vi "Lab Panel V5.25.1.vi"() -> ()   [LabVIEW 2013] (continued)
                    n2215 = Unbundle By Name(w3901) -> ("1  (A) cal"=w3894:dbl, "1 (V) cal"=w3893:dbl, "1 (PF) cal"=w3892:dbl, "2 (A) cal"=w3891:dbl, "2 (V) cal"=w3890:dbl, "2 (PF) cal"=w3889:dbl)  [unwired: 4 out]
                    n2216 = Multiply(x=w3900, y=w3894) -> (x*y=w3887:dbl)
                    n2217 = Multiply(x=w3899, y=w3893) -> (x*y=w3881:dbl)
                    n2218 = Multiply(x=w3898, y=w3892) -> (x*y=w3886:dbl)
                    n2219 = Multiply(x=w3897, y=w3891) -> (x*y=w3884:dbl)
                    n2220 = Multiply(x=w3896, y=w3890) -> (x*y=w3883:dbl)
                    n2221 = Multiply(x=w3895, y=w3889) -> (x*y=w3882:dbl)
                    n2222 = local read "SIG LAB03-1"() -> (w3888:T2)
                    n2223 = local read "SIG LAB03-2"() -> (w3885:T2)
                    n2224 = Bundle By Name(cluster=w3888, "AMPS"=w3887, "VOLTS"=w3881, "PF"=w3886) -> (w3880:T2)
                    n2225 = Bundle By Name(cluster=w3885, "AMPS"=w3884, "VOLTS"=w3883, "PF"=w3882) -> (w3879:T2)
                    n2226 = global write "Global display 1.vi" "SIG LAB03-1"(w3880) -> ()
                    n2227 = global write "Global display 1.vi" "SIG LAB03-2"(w3879) -> ()
                    n2228 = local write "SIG LAB03-2"(w3879) -> ()
                    n2229 = local write "SIG LAB03-1"(w3880) -> ()
                  }
                  frame #5 {
                    n2230 = case shown="False" w3931 {
                      tunnel: [w3933 w3934] -> w3929
                      tunnel: w3930 -> [_ w3934]
                      frame False {
                        n2231 = local read "CAL LAB04"() -> (w3933:T14)
                      }
                      frame True {
                      }
                    }
                    n2232 = Unbundle By Name(w3932) -> ("OFF amps"=w3928:dbl, "VOLTS"=w3927:dbl, "PF"=w3926:dbl, "OFF amps"=w3925:dbl, "VOLTS"=w3924:dbl, "PF"=w3923:dbl)
                    n2233 = Unbundle By Name(w3929) -> ("1  (A) cal"=w3922:dbl, "1 (V) cal"=w3921:dbl, "1 (PF) cal"=w3920:dbl, "2 (A) cal"=w3919:dbl, "2 (V) cal"=w3918:dbl, "2 (PF) cal"=w3917:dbl)  [unwired: 4 out]
                    n2234 = Multiply(x=w3928, y=w3922) -> (x*y=w3915:dbl)
                    n2235 = Multiply(x=w3927, y=w3921) -> (x*y=w3914:dbl)
                    n2236 = Multiply(x=w3926, y=w3920) -> (x*y=w3913:dbl)
                    n2237 = Multiply(x=w3925, y=w3919) -> (x*y=w3911:dbl)
                    n2238 = Multiply(x=w3924, y=w3918) -> (x*y=w3910:dbl)
                    n2239 = Multiply(x=w3923, y=w3917) -> (x*y=w3909:dbl)
                    n2240 = local read "SIG LAB04-1"() -> (w3916:T2)
                    n2241 = local read "SIG LAB04-2"() -> (w3912:T2)
                    n2242 = Bundle By Name(cluster=w3916, "AMPS"=w3915, "VOLTS"=w3914, "PF"=w3913) -> (w3908:T2)
                    n2243 = Bundle By Name(cluster=w3912, "AMPS"=w3911, "VOLTS"=w3910, "PF"=w3909) -> (w3907:T2)
                    n2244 = global write "Global display 1.vi" "SIG LAB04-2"(w3907) -> ()
                    n2245 = global write "Global display 1.vi" "SIG LAB04-1"(w3908) -> ()
                    n2246 = local write "SIG LAB04-2"(w3907) -> ()
                    n2247 = local write "SIG LAB04-1"(w3908) -> ()
                  }
                  frame #6 {
                    n2248 = Unbundle By Name(w3960) -> ("OFF amps"=w3956:dbl, "VOLTS"=w3937:dbl, "PF"=w3955:dbl, "OFF amps"=w3954:dbl, "VOLTS"=w3953:dbl, "PF"=w3952:dbl)
                    n2249 = case shown="False" w3959 {
                      tunnel: [w3961 w3962] -> w3957
                      tunnel: w3958 -> [_ w3962]
                      frame False {
                        n2250 = local read "CAL LAB05"() -> (w3961:T14)
                      }
                      frame True {
                      }
                    }
                    n2251 = Unbundle By Name(w3957) -> ("1  (A) cal"=w3951:dbl, "1 (V) cal"=w3950:dbl, "1 (PF) cal"=w3949:dbl, "2 (A) cal"=w3948:dbl, "2 (V) cal"=w3947:dbl, "2 (PF) cal"=w3946:dbl)  [unwired: 4 out]
                    n2252 = Multiply(x=w3956, y=w3951) -> (x*y=w3944:dbl)
                    n2253 = Multiply(x=w3937, y=w3950) -> (x*y=w3943:dbl)
                    n2254 = Multiply(x=w3955, y=w3949) -> (x*y=w3942:dbl)
                    n2255 = Multiply(x=w3954, y=w3948) -> (x*y=w3940:dbl)
                    n2256 = Multiply(x=w3953, y=w3947) -> (x*y=w3939:dbl)
                    n2257 = Multiply(x=w3952, y=w3946) -> (x*y=w3938:dbl)
                    n2258 = local read "SIG LAB05-1"() -> (w3945:T2)
                    n2259 = local read "SIG LAB05-2"() -> (w3941:T2)
                    n2260 = Bundle By Name(cluster=w3945, "AMPS"=w3944, "VOLTS"=w3943, "PF"=w3942) -> (w3936:T2)
                    n2261 = Bundle By Name(cluster=w3941, "AMPS"=w3940, "VOLTS"=w3939, "PF"=w3938) -> (w3935:T2)
                    n2262 = global write "Global display 1.vi" "SIG LAB05-1"(w3936) -> ()
                    n2263 = global write "Global display 1.vi" "SIG LAB05-2"(w3935) -> ()
                    n2264 = local write "SIG LAB05-2"(w3935) -> ()
                    n2265 = local write "SIG LAB05-1"(w3936) -> ()
                  }
                  frame #7 {
                    n2266 = case shown="False" w3963 {
                      tunnel: w3965 -> [w3970 _]
                      tunnel: w3964 -> [w3969 _]
                      frame False {
                        # "update ambient referance temperature"
                        n2267 = case shown="True" w3970 {
                          tunnel: [w3972 100.0] -> w3971
                          frame False {
                            n2268 = local read "TEMP REF cal"() -> (w3972:dbl)
                          }
                          frame True {
                          }
                        }
                        n2269 = disable-structure shown="Disabled" {
                          frame Disabled {
                            n2270 = local read "Temp read loop"() -> ()  [unwired: 1 out]
                          }
                          frame Enabled {
                          }
                        }
                        n2271 = Multiply(x=w3971, y=w3969) -> (x*y=w3968:dbl)
                        n2272 = Subtract(x=w3968, y=272) -> (x-y=w3966:dbl)
                        "Amb Tp" <- w3966
                        n2273 = local write "Ref deg C"(w3966) -> ()
                        "deg C (volts)" <- w3969
                      }
                      frame True {
                      }
                    }
                  }
                }
              }
            }
          }
          frame #14 {
            # "save test data to file"
            n2274 = local read "on loops"() -> (w3993:dbl)
            n2275 = Get Date/Time In Seconds() -> (seconds since 1Jan1904=w3974:timestamp)
            "File Time Stamp" <- w3974
            n2276 = local read "jig cycle"() -> (w3990:dbl)
            n2277 = Format Date/Time String(time format string (%c)="%H:%M%:%S", seconds (now)=w3974) -> (date/time string=w3978:string)  [unwired: 1 in]
            n2278 = Add(x=w3993, y=4) -> (x+y=w3991:dbl)
            n2279 = Build Array(w3978) -> (w3977:string[])
            n2280 = Equal?(x=w3990, y=3) -> (x = y?=w3976:bool)
            n2281 = Equal?(x=w3990, y=w3991) -> (x = y?=w3975:bool)
            n2282 = stacked-sequence {
              tunnel: w3989 -> [w3999 _ _ _ _ _ _ _ _ _]
              tunnel: w3988 -> [_ w4075 _ _ _ _ _ _ _ _]
              tunnel: w3987 -> [_ _ w4155 _ _ _ _ _ _ _]
              tunnel: w3986 -> [_ _ _ w4235 _ _ _ _ _ _]
              tunnel: w3985 -> [_ _ _ _ w4315 _ _ _ _ _]
              tunnel: w3984 -> [_ _ _ _ _ w4395 _ _ _ _]
              tunnel: w3983 -> [_ _ _ _ _ _ w4475 _ _ _]
              tunnel: w3982 -> [_ _ _ _ _ _ _ w4555 _ _]
              tunnel: w3981 -> [_ _ _ _ _ _ _ _ w4635 _]
              tunnel: w3980 -> [_ _ _ _ _ _ _ _ _ w4715]
              tunnel: w3977 -> [w3998 w4079 w4159 w4239 w4319 w4399 w4479 w4559 w4639 w4719]
              tunnel: w3976 -> [w3997 w4078 w4158 w4238 w4318 w4398 w4478 w4558 w4638 w4718]
              tunnel: w3975 -> [w3996 w4077 w4157 w4237 w4317 w4397 w4477 w4557 w4637 w4717]
              tunnel: w3974 -> [w3995 w4076 w4156 w4236 w4316 w4396 w4476 w4556 w4636 w4716]
              frame #0 {
                n2283 = case shown="True" w3999 {
                  tunnel: w3998 -> [_ w4004]
                  tunnel: w3997 -> [_ w4003]
                  tunnel: w3996 -> [_ w4001]
                  tunnel: w3995 -> [_ w4000]
                  frame False {
                  }
                  frame True {
                    n2284 = local read "DISP LAB01-1"() -> (w4005:T4)
                    n2285 = local read "SIG LAB01-1"() -> (w4006:T2)
                    n2286 = local read "ON L01-1"() -> (w4002:cluster{"amps":dbl, "volts":dbl, "pf":dbl})
                    n2287 = Unbundle(w4006) -> ("AMPS"=w4012:dbl, "VOLTS"=w4010:dbl, "PF"=w4009:dbl, "Tmp Live"=w4008:dbl, "Tmp Neut"=w4011:dbl)
                    n2288 = Unbundle(w4005) -> ("CYCLE"=w4007:dbl)  [unwired: 2 out]
                    n2289 = stacked-sequence {
                      tunnel: w4012 -> [w4016 w4035]
                      tunnel: w4011 -> [_ w4034]
                      tunnel: w4010 -> [w4015 w4033]
                      tunnel: w4009 -> [w4014 w4032]
                      tunnel: w4008 -> [_ w4031]
                      tunnel: w4007 -> [_ w4030]
                      tunnel: w4004 -> [_ w4029]
                      tunnel: w4003 -> [w4017 _]
                      tunnel: w4002 -> [w4013 w4027]
                      tunnel: w4001 -> [_ w4028]
                      tunnel: w4000 -> [_ w4023]
                      frame #0 {
                        n2290 = case shown="True" w4017 {
                          tunnel: w4016 -> [_ w4022]
                          tunnel: w4015 -> [_ w4021]
                          tunnel: w4014 -> [_ w4020]
                          tunnel: w4013 -> [_ w4018]
                          frame False {
                          }
                          frame True {
                            n2291 = Bundle(cluster=w4018, "amps"=w4022, "volts"=w4021, "pf"=w4020) -> (w4019:cluster{"amps":dbl, "volts":dbl, "pf":dbl})
                            n2292 = local write "ON L01-1"(w4019) -> ()
                          }
                        }
                      }
                      frame #1 {
                        n2293 = Unbundle(w4027) -> ("amps"=w4026:dbl, "volts"=w4025:dbl, "pf"=w4024:dbl)
                        n2294 = case shown="True" w4028 {
                          tunnel: w4035 -> [_ w4036]
                          tunnel: w4034 -> [_ w4074]
                          tunnel: w4033 -> [_ _]
                          tunnel: w4032 -> [_ _]
                          tunnel: w4031 -> [_ w4073]
                          tunnel: w4030 -> [_ w4072]
                          tunnel: w4029 -> [_ w4040]
                          tunnel: w4026 -> [_ w4037]
                          tunnel: w4025 -> [_ w4069]
                          tunnel: w4024 -> [_ w4068]
                          tunnel: w4023 -> [_ w4038]
                          frame False {
                          }
                          frame True {
                            n2295 = local read "TDMS LAB01-1"() -> (w4071:refnum<k34>)
                            n2296 = Build Array(w4069) -> (w4065:dbl[])
                            n2297 = Build Array(w4068) -> (w4064:dbl[])
                            n2298 = Build Array(w4073) -> (w4063:dbl[])
                            n2299 = Build Array(w4074) -> (w4062:dbl[])
                            n2300 = Build Array(w4037) -> (w4067:dbl[])
                            n2301 = Build Array(w4036) -> (w4066:dbl[])
                            n2302 = Build Array(w4072) -> (w4061:dbl[])
                            n2303 = Build Array("AMPS ON", "AMPS OFF", "VOLTS", "PF", "TEMP Live", "TEMP Neut", "CYCLE") -> (w4045:string[])
                            n2304 = Bundle By Name("Y"=w4067, "t0"=w4038) -> (w4060:waveform(dbl))  [unwired: 1 in]
                            n2305 = Bundle By Name("Y"=w4066, "t0"=w4038) -> (w4059:waveform(dbl))  [unwired: 1 in]
                            n2306 = Bundle By Name("Y"=w4065, "t0"=w4038) -> (w4058:waveform(dbl))  [unwired: 1 in]
                            n2307 = Bundle By Name("Y"=w4064, "t0"=w4038) -> (w4057:waveform(dbl))  [unwired: 1 in]
                            n2308 = Bundle By Name("Y"=w4063, "t0"=w4038) -> (w4056:waveform(dbl))  [unwired: 1 in]
                            n2309 = Bundle By Name("Y"=w4062, "t0"=w4038) -> (w4055:waveform(dbl))  [unwired: 1 in]
                            n2310 = Bundle By Name("Y"=w4061, "t0"=w4038) -> (w4054:waveform(dbl))  [unwired: 1 in]
                            n2311 = Build Array(w4060, w4059, w4058, w4057, w4056, w4055, w4054) -> (w4053:waveform(dbl)[])
                            n2312 = TDMS Write(0:w4071, 5:"TEST VALUES", 7:w4045, 9:w4053) -> (4:w4044:refnum<k34>, 6:w4043:string, 15:w4042:errorcluster)  [unwired: 2 in, 1 out]
                            n2313 = TDMS Write(0:w4044, 5:w4043, 7:"TIME", 9:w4040, 11:w4042) -> (15:w4039:errorcluster)  [unwired: 1 in, 3 out]
                            n2314 = local write "data file error"(w4039) -> ()
                          }
                        }
                      }
                    }
                  }
                }
              }
              frame #1 {
                n2315 = case shown="True" w4075 {
                  tunnel: w4079 -> [_ w4084]
                  tunnel: w4078 -> [_ w4083]
                  tunnel: w4077 -> [_ w4081]
                  tunnel: w4076 -> [_ w4080]
                  frame False {
                  }
                  frame True {
                    n2316 = local read "DISP LAB01-2"() -> (w4085:T4)
                    n2317 = local read "SIG LAB01-2"() -> (w4086:T2)
                    n2318 = local read "ON L01-2"() -> (w4082:cluster{"amps":dbl, "volts":dbl, "pf":dbl})
                    n2319 = Unbundle(w4086) -> ("AMPS"=w4092:dbl, "VOLTS"=w4090:dbl, "PF"=w4089:dbl, "Tmp Live"=w4088:dbl, "Tmp Neut"=w4091:dbl)
                    n2320 = Unbundle(w4085) -> ("CYCLE"=w4087:dbl)  [unwired: 2 out]
                    n2321 = stacked-sequence {
                      tunnel: w4092 -> [w4096 w4115]
                      tunnel: w4091 -> [_ w4114]
                      tunnel: w4090 -> [w4095 w4113]
                      tunnel: w4089 -> [w4094 w4112]
                      tunnel: w4088 -> [_ w4111]
                      tunnel: w4087 -> [_ w4110]
                      tunnel: w4084 -> [_ w4109]
                      tunnel: w4083 -> [w4097 _]
                      tunnel: w4082 -> [w4093 w4107]
                      tunnel: w4081 -> [_ w4108]
                      tunnel: w4080 -> [_ w4103]
                      frame #0 {
                        n2322 = case shown="True" w4097 {
                          tunnel: w4096 -> [_ w4102]
                          tunnel: w4095 -> [_ w4101]
                          tunnel: w4094 -> [_ w4100]
                          tunnel: w4093 -> [_ w4098]
                          frame False {
                          }
                          frame True {
                            n2323 = Bundle(cluster=w4098, "amps"=w4102, "volts"=w4101, "pf"=w4100) -> (w4099:cluster{"amps":dbl, "volts":dbl, "pf":dbl})
                            n2324 = local write "ON L01-2"(w4099) -> ()
                          }
                        }
                      }
                      frame #1 {
                        n2325 = Unbundle(w4107) -> ("amps"=w4106:dbl, "volts"=w4105:dbl, "pf"=w4104:dbl)
                        n2326 = case shown="True" w4108 {
                          tunnel: w4115 -> [_ w4147]
                          tunnel: w4114 -> [_ w4154]
                          tunnel: w4113 -> [_ _]
                          tunnel: w4112 -> [_ _]
                          tunnel: w4111 -> [_ w4153]
                          tunnel: w4110 -> [_ w4152]
                          tunnel: w4109 -> [_ w4117]
                          tunnel: w4106 -> [_ w4149]
                          tunnel: w4105 -> [_ w4148]
                          tunnel: w4104 -> [_ w4146]
                          tunnel: w4103 -> [_ w4138]
                          frame False {
                          }
                          frame True {
                            n2327 = local read "TDMS LAB01-2"() -> (w4151:refnum<k34>)
                            n2328 = Build Array(w4148) -> (w4143:dbl[])
                            n2329 = Build Array(w4146) -> (w4142:dbl[])
                            n2330 = Build Array(w4153) -> (w4141:dbl[])
                            n2331 = Build Array(w4154) -> (w4140:dbl[])
                            n2332 = Build Array(w4149) -> (w4145:dbl[])
                            n2333 = Build Array(w4147) -> (w4144:dbl[])
                            n2334 = Build Array(w4152) -> (w4139:dbl[])
                            n2335 = Build Array("AMPS ON", "AMPS OFF", "VOLTS", "PF", "TEMP Live", "TEMP Neut", "CYCLE") -> (w4122:string[])
                            n2336 = Bundle By Name("Y"=w4145, "t0"=w4138) -> (w4137:waveform(dbl))  [unwired: 1 in]
                            n2337 = Bundle By Name("Y"=w4144, "t0"=w4138) -> (w4136:waveform(dbl))  [unwired: 1 in]
                            n2338 = Bundle By Name("Y"=w4143, "t0"=w4138) -> (w4135:waveform(dbl))  [unwired: 1 in]
                            n2339 = Bundle By Name("Y"=w4142, "t0"=w4138) -> (w4134:waveform(dbl))  [unwired: 1 in]
                            n2340 = Bundle By Name("Y"=w4141, "t0"=w4138) -> (w4133:waveform(dbl))  [unwired: 1 in]
                            n2341 = Bundle By Name("Y"=w4140, "t0"=w4138) -> (w4132:waveform(dbl))  [unwired: 1 in]
                            n2342 = Bundle By Name("Y"=w4139, "t0"=w4138) -> (w4131:waveform(dbl))  [unwired: 1 in]
                            n2343 = Build Array(w4137, w4136, w4135, w4134, w4133, w4132, w4131) -> (w4130:waveform(dbl)[])
                            n2344 = TDMS Write(0:w4151, 5:"TEST VALUES", 7:w4122, 9:w4130) -> (4:w4121:refnum<k34>, 6:w4120:string, 15:w4119:errorcluster)  [unwired: 2 in, 1 out]
                            n2345 = TDMS Write(0:w4121, 5:w4120, 7:"TIME", 9:w4117, 11:w4119) -> (15:w4116:errorcluster)  [unwired: 1 in, 3 out]
                            n2346 = local write "data file error"(w4116) -> ()
                          }
                        }
                      }
                    }
                  }
                }
              }
              frame #2 {
                n2347 = case shown="True" w4155 {
                  tunnel: w4159 -> [_ w4164]
                  tunnel: w4158 -> [_ w4163]
                  tunnel: w4157 -> [_ w4161]
                  tunnel: w4156 -> [_ w4160]
                  frame False {
                  }
                  frame True {
                    n2348 = local read "DISP LAB02-1"() -> (w4165:T4)
                    n2349 = local read "SIG LAB02-1"() -> (w4166:T2)
                    n2350 = local read "ON L02-1"() -> (w4162:cluster{"amps":dbl, "volts":dbl, "pf":dbl})
                    n2351 = Unbundle(w4166) -> ("AMPS"=w4172:dbl, "VOLTS"=w4170:dbl, "PF"=w4169:dbl, "Tmp Live"=w4168:dbl, "Tmp Neut"=w4171:dbl)
                    n2352 = Unbundle(w4165) -> ("CYCLE"=w4167:dbl)  [unwired: 2 out]
                    n2353 = stacked-sequence {
                      tunnel: w4172 -> [w4176 w4195]
                      tunnel: w4171 -> [_ w4194]
                      tunnel: w4170 -> [w4175 w4193]
                      tunnel: w4169 -> [w4174 w4192]
                      tunnel: w4168 -> [_ w4191]
                      tunnel: w4167 -> [_ w4190]
                      tunnel: w4164 -> [_ w4189]
                      tunnel: w4163 -> [w4177 _]
                      tunnel: w4162 -> [w4173 w4187]
                      tunnel: w4161 -> [_ w4188]
                      tunnel: w4160 -> [_ w4183]
                      frame #0 {
                        n2354 = case shown="True" w4177 {
                          tunnel: w4176 -> [_ w4182]
                          tunnel: w4175 -> [_ w4181]
                          tunnel: w4174 -> [_ w4180]
                          tunnel: w4173 -> [_ w4178]
                          frame False {
                          }
                          frame True {
                            n2355 = Bundle(cluster=w4178, "amps"=w4182, "volts"=w4181, "pf"=w4180) -> (w4179:cluster{"amps":dbl, "volts":dbl, "pf":dbl})
                            n2356 = local write "ON L02-1"(w4179) -> ()
                          }
                        }
                      }
                      frame #1 {
                        n2357 = Unbundle(w4187) -> ("amps"=w4186:dbl, "volts"=w4185:dbl, "pf"=w4184:dbl)
                        n2358 = case shown="True" w4188 {
                          tunnel: w4195 -> [_ w4227]
                          tunnel: w4194 -> [_ w4234]
                          tunnel: w4193 -> [_ _]
                          tunnel: w4192 -> [_ _]
                          tunnel: w4191 -> [_ w4233]
                          tunnel: w4190 -> [_ w4232]
                          tunnel: w4189 -> [_ w4197]
                          tunnel: w4186 -> [_ w4229]
                          tunnel: w4185 -> [_ w4228]
                          tunnel: w4184 -> [_ w4226]
                          tunnel: w4183 -> [_ w4218]
                          frame False {
                          }
                          frame True {
                            n2359 = local read "TDMS LAB02-1"() -> (w4231:refnum<k34>)
                            n2360 = Build Array(w4228) -> (w4223:dbl[])
                            n2361 = Build Array(w4226) -> (w4222:dbl[])
                            n2362 = Build Array(w4233) -> (w4221:dbl[])
                            n2363 = Build Array(w4234) -> (w4220:dbl[])
                            n2364 = Build Array(w4229) -> (w4225:dbl[])
                            n2365 = Build Array(w4227) -> (w4224:dbl[])
                            n2366 = Build Array(w4232) -> (w4219:dbl[])
                            n2367 = Build Array("AMPS ON", "AMPS OFF", "VOLTS", "PF", "TEMP Live", "TEMP Neut", "CYCLE") -> (w4202:string[])
                            n2368 = Bundle By Name("Y"=w4225, "t0"=w4218) -> (w4217:waveform(dbl))  [unwired: 1 in]
                            n2369 = Bundle By Name("Y"=w4224, "t0"=w4218) -> (w4216:waveform(dbl))  [unwired: 1 in]
                            n2370 = Bundle By Name("Y"=w4223, "t0"=w4218) -> (w4215:waveform(dbl))  [unwired: 1 in]
                            n2371 = Bundle By Name("Y"=w4222, "t0"=w4218) -> (w4214:waveform(dbl))  [unwired: 1 in]
                            n2372 = Bundle By Name("Y"=w4221, "t0"=w4218) -> (w4213:waveform(dbl))  [unwired: 1 in]
                            n2373 = Bundle By Name("Y"=w4220, "t0"=w4218) -> (w4212:waveform(dbl))  [unwired: 1 in]
                            n2374 = Bundle By Name("Y"=w4219, "t0"=w4218) -> (w4211:waveform(dbl))  [unwired: 1 in]
                            n2375 = Build Array(w4217, w4216, w4215, w4214, w4213, w4212, w4211) -> (w4210:waveform(dbl)[])
                            n2376 = TDMS Write(0:w4231, 5:"TEST VALUES", 7:w4202, 9:w4210) -> (4:w4201:refnum<k34>, 6:w4200:string, 15:w4199:errorcluster)  [unwired: 2 in, 1 out]
                            n2377 = TDMS Write(0:w4201, 5:w4200, 7:"TIME", 9:w4197, 11:w4199) -> (15:w4196:errorcluster)  [unwired: 1 in, 3 out]
                            n2378 = local write "data file error"(w4196) -> ()
                          }
                        }
                      }
                    }
                  }
                }
              }
              frame #3 {
                n2379 = case shown="True" w4235 {
                  tunnel: w4239 -> [_ w4244]
                  tunnel: w4238 -> [_ w4243]
                  tunnel: w4237 -> [_ w4241]
                  tunnel: w4236 -> [_ w4240]
                  frame False {
                  }
                  frame True {
                    n2380 = local read "DISP LAB02-2"() -> (w4245:T4)
                    n2381 = local read "SIG LAB02-2"() -> (w4246:T2)
                    n2382 = local read "ON L02-2"() -> (w4242:cluster{"amps":dbl, "volts":dbl, "pf":dbl})
                    n2383 = Unbundle(w4246) -> ("AMPS"=w4252:dbl, "VOLTS"=w4250:dbl, "PF"=w4249:dbl, "Tmp Live"=w4248:dbl, "Tmp Neut"=w4251:dbl)
                    n2384 = Unbundle(w4245) -> ("CYCLE"=w4247:dbl)  [unwired: 2 out]
                    n2385 = stacked-sequence {
                      tunnel: w4252 -> [w4256 w4275]
                      tunnel: w4251 -> [_ w4274]
                      tunnel: w4250 -> [w4255 w4273]
                      tunnel: w4249 -> [w4254 w4272]
                      tunnel: w4248 -> [_ w4271]
                      tunnel: w4247 -> [_ w4270]
                      tunnel: w4244 -> [_ w4269]
                      tunnel: w4243 -> [w4257 _]
                      tunnel: w4242 -> [w4253 w4267]
                      tunnel: w4241 -> [_ w4268]
                      tunnel: w4240 -> [_ w4263]
                      frame #0 {
                        n2386 = case shown="True" w4257 {
                          tunnel: w4256 -> [_ w4262]
                          tunnel: w4255 -> [_ w4261]
                          tunnel: w4254 -> [_ w4260]
                          tunnel: w4253 -> [_ w4258]
                          frame False {
                          }
                          frame True {
                            n2387 = Bundle(cluster=w4258, "amps"=w4262, "volts"=w4261, "pf"=w4260) -> (w4259:cluster{"amps":dbl, "volts":dbl, "pf":dbl})
                            n2388 = local write "ON L02-2"(w4259) -> ()
                          }
                        }
                      }
                      frame #1 {
                        n2389 = Unbundle(w4267) -> ("amps"=w4266:dbl, "volts"=w4265:dbl, "pf"=w4264:dbl)
                        n2390 = case shown="True" w4268 {
                          tunnel: w4275 -> [_ w4307]
                          tunnel: w4274 -> [_ w4314]
                          tunnel: w4273 -> [_ _]
                          tunnel: w4272 -> [_ _]
                          tunnel: w4271 -> [_ w4313]
                          tunnel: w4270 -> [_ w4312]
                          tunnel: w4269 -> [_ w4277]
                          tunnel: w4266 -> [_ w4309]
                          tunnel: w4265 -> [_ w4308]
                          tunnel: w4264 -> [_ w4306]
                          tunnel: w4263 -> [_ w4298]
                          frame False {
                          }
                          frame True {
                            n2391 = local read "TDMS LAB02-2"() -> (w4311:refnum<k34>)
                            n2392 = Build Array(w4308) -> (w4303:dbl[])
                            n2393 = Build Array(w4306) -> (w4302:dbl[])
                            n2394 = Build Array(w4313) -> (w4301:dbl[])
                            n2395 = Build Array(w4314) -> (w4300:dbl[])
                            n2396 = Build Array(w4309) -> (w4305:dbl[])
                            n2397 = Build Array(w4307) -> (w4304:dbl[])
                            n2398 = Build Array(w4312) -> (w4299:dbl[])
                            n2399 = Build Array("AMPS ON", "AMPS OFF", "VOLTS", "PF", "TEMP Live", "TEMP Neut", "CYCLE") -> (w4282:string[])
                            n2400 = Bundle By Name("Y"=w4305, "t0"=w4298) -> (w4297:waveform(dbl))  [unwired: 1 in]
                            n2401 = Bundle By Name("Y"=w4304, "t0"=w4298) -> (w4296:waveform(dbl))  [unwired: 1 in]
                            n2402 = Bundle By Name("Y"=w4303, "t0"=w4298) -> (w4295:waveform(dbl))  [unwired: 1 in]
                            n2403 = Bundle By Name("Y"=w4302, "t0"=w4298) -> (w4294:waveform(dbl))  [unwired: 1 in]
                            n2404 = Bundle By Name("Y"=w4301, "t0"=w4298) -> (w4293:waveform(dbl))  [unwired: 1 in]
                            n2405 = Bundle By Name("Y"=w4300, "t0"=w4298) -> (w4292:waveform(dbl))  [unwired: 1 in]
                            n2406 = Bundle By Name("Y"=w4299, "t0"=w4298) -> (w4291:waveform(dbl))  [unwired: 1 in]
                            n2407 = Build Array(w4297, w4296, w4295, w4294, w4293, w4292, w4291) -> (w4290:waveform(dbl)[])
                            n2408 = TDMS Write(0:w4311, 5:"TEST VALUES", 7:w4282, 9:w4290) -> (4:w4281:refnum<k34>, 6:w4280:string, 15:w4279:errorcluster)  [unwired: 2 in, 1 out]
                            n2409 = TDMS Write(0:w4281, 5:w4280, 7:"TIME", 9:w4277, 11:w4279) -> (15:w4276:errorcluster)  [unwired: 1 in, 3 out]
                            n2410 = local write "data file error"(w4276) -> ()
                          }
                        }
                      }
                    }
                  }
                }
              }
              frame #4 {
                n2411 = case shown="True" w4315 {
                  tunnel: w4319 -> [_ w4324]
                  tunnel: w4318 -> [_ w4323]
                  tunnel: w4317 -> [_ w4321]
                  tunnel: w4316 -> [_ w4320]
                  frame False {
                  }
                  frame True {
                    n2412 = local read "DISP LAB03-1"() -> (w4325:T4)
                    n2413 = local read "SIG LAB03-1"() -> (w4326:T2)
                    n2414 = local read "ON L03-1"() -> (w4322:cluster{"amps":dbl, "volts":dbl, "pf":dbl})
                    n2415 = Unbundle(w4326) -> ("AMPS"=w4332:dbl, "VOLTS"=w4330:dbl, "PF"=w4329:dbl, "Tmp Live"=w4328:dbl, "Tmp Neut"=w4331:dbl)
                    n2416 = Unbundle(w4325) -> ("CYCLE"=w4327:dbl)  [unwired: 2 out]
                    n2417 = stacked-sequence {
                      tunnel: w4332 -> [w4336 w4355]
                      tunnel: w4331 -> [_ w4354]
                      tunnel: w4330 -> [w4335 w4353]
                      tunnel: w4329 -> [w4334 w4352]
                      tunnel: w4328 -> [_ w4351]
                      tunnel: w4327 -> [_ w4350]
                      tunnel: w4324 -> [_ w4349]
                      tunnel: w4323 -> [w4337 _]
                      tunnel: w4322 -> [w4333 w4347]
                      tunnel: w4321 -> [_ w4348]
                      tunnel: w4320 -> [_ w4343]
                      frame #0 {
                        n2418 = case shown="True" w4337 {
                          tunnel: w4336 -> [_ w4342]
                          tunnel: w4335 -> [_ w4341]
                          tunnel: w4334 -> [_ w4340]
                          tunnel: w4333 -> [_ w4338]
                          frame False {
                          }
                          frame True {
                            n2419 = Bundle(cluster=w4338, "amps"=w4342, "volts"=w4341, "pf"=w4340) -> (w4339:cluster{"amps":dbl, "volts":dbl, "pf":dbl})
                            n2420 = local write "ON L03-1"(w4339) -> ()
                          }
                        }
                      }
                      frame #1 {
                        n2421 = Unbundle(w4347) -> ("amps"=w4346:dbl, "volts"=w4345:dbl, "pf"=w4344:dbl)
                        n2422 = case shown="True" w4348 {
                          tunnel: w4355 -> [_ w4387]
                          tunnel: w4354 -> [_ w4394]
                          tunnel: w4353 -> [_ _]
                          tunnel: w4352 -> [_ _]
                          tunnel: w4351 -> [_ w4393]
                          tunnel: w4350 -> [_ w4392]
                          tunnel: w4349 -> [_ w4357]
                          tunnel: w4346 -> [_ w4389]
                          tunnel: w4345 -> [_ w4388]
                          tunnel: w4344 -> [_ w4386]
                          tunnel: w4343 -> [_ w4378]
                          frame False {
                          }
                          frame True {
                            n2423 = local read "TDMS LAB03-1"() -> (w4391:refnum<k34>)
                            n2424 = Build Array(w4388) -> (w4383:dbl[])
                            n2425 = Build Array(w4386) -> (w4382:dbl[])
                            n2426 = Build Array(w4393) -> (w4381:dbl[])
                            n2427 = Build Array(w4394) -> (w4380:dbl[])
                            n2428 = Build Array(w4389) -> (w4385:dbl[])
                            n2429 = Build Array(w4387) -> (w4384:dbl[])
                            n2430 = Build Array(w4392) -> (w4379:dbl[])
                            n2431 = Build Array("AMPS ON", "AMPS OFF", "VOLTS", "PF", "TEMP Live", "TEMP Neut", "CYCLE") -> (w4362:string[])
                            n2432 = Bundle By Name("Y"=w4385, "t0"=w4378) -> (w4377:waveform(dbl))  [unwired: 1 in]
                            n2433 = Bundle By Name("Y"=w4384, "t0"=w4378) -> (w4376:waveform(dbl))  [unwired: 1 in]
                            n2434 = Bundle By Name("Y"=w4383, "t0"=w4378) -> (w4375:waveform(dbl))  [unwired: 1 in]
                            n2435 = Bundle By Name("Y"=w4382, "t0"=w4378) -> (w4374:waveform(dbl))  [unwired: 1 in]
                            n2436 = Bundle By Name("Y"=w4381, "t0"=w4378) -> (w4373:waveform(dbl))  [unwired: 1 in]
                            n2437 = Bundle By Name("Y"=w4380, "t0"=w4378) -> (w4372:waveform(dbl))  [unwired: 1 in]
                            n2438 = Bundle By Name("Y"=w4379, "t0"=w4378) -> (w4371:waveform(dbl))  [unwired: 1 in]
                            n2439 = Build Array(w4377, w4376, w4375, w4374, w4373, w4372, w4371) -> (w4370:waveform(dbl)[])
                            n2440 = TDMS Write(0:w4391, 5:"TEST VALUES", 7:w4362, 9:w4370) -> (4:w4361:refnum<k34>, 6:w4360:string, 15:w4359:errorcluster)  [unwired: 2 in, 1 out]
                            n2441 = TDMS Write(0:w4361, 5:w4360, 7:"TIME", 9:w4357, 11:w4359) -> (15:w4356:errorcluster)  [unwired: 1 in, 3 out]
                            n2442 = local write "data file error"(w4356) -> ()
                          }
                        }
                      }
                    }
                  }
                }
              }
              frame #5 {
                n2443 = case shown="True" w4395 {
                  tunnel: w4399 -> [_ w4404]
                  tunnel: w4398 -> [_ w4403]
                  tunnel: w4397 -> [_ w4401]
                  tunnel: w4396 -> [_ w4400]
                  frame False {
                  }
                  frame True {
                    n2444 = local read "DISP LAB03-2"() -> (w4405:T4)
                    n2445 = local read "SIG LAB03-2"() -> (w4406:T2)
                    n2446 = local read "ON L03-2"() -> (w4402:cluster{"amps":dbl, "volts":dbl, "pf":dbl})
                    n2447 = Unbundle(w4406) -> ("AMPS"=w4412:dbl, "VOLTS"=w4410:dbl, "PF"=w4409:dbl, "Tmp Live"=w4408:dbl, "Tmp Neut"=w4411:dbl)
                    n2448 = Unbundle(w4405) -> ("CYCLE"=w4407:dbl)  [unwired: 2 out]
                    n2449 = stacked-sequence {
                      tunnel: w4412 -> [w4416 w4435]
                      tunnel: w4411 -> [_ w4434]
                      tunnel: w4410 -> [w4415 w4433]
                      tunnel: w4409 -> [w4414 w4432]
                      tunnel: w4408 -> [_ w4431]
                      tunnel: w4407 -> [_ w4430]
                      tunnel: w4404 -> [_ w4429]
                      tunnel: w4403 -> [w4417 _]
                      tunnel: w4402 -> [w4413 w4427]
                      tunnel: w4401 -> [_ w4428]
                      tunnel: w4400 -> [_ w4423]
                      frame #0 {
                        n2450 = case shown="True" w4417 {
                          tunnel: w4416 -> [_ w4422]
                          tunnel: w4415 -> [_ w4421]
                          tunnel: w4414 -> [_ w4420]
                          tunnel: w4413 -> [_ w4418]
                          frame False {
                          }
                          frame True {
                            n2451 = Bundle(cluster=w4418, "amps"=w4422, "volts"=w4421, "pf"=w4420) -> (w4419:cluster{"amps":dbl, "volts":dbl, "pf":dbl})
                            n2452 = local write "ON L03-2"(w4419) -> ()
                          }
                        }
                      }
                      frame #1 {
                        n2453 = Unbundle(w4427) -> ("amps"=w4426:dbl, "volts"=w4425:dbl, "pf"=w4424:dbl)
                        n2454 = case shown="True" w4428 {
                          tunnel: w4435 -> [_ w4467]
                          tunnel: w4434 -> [_ w4474]
                          tunnel: w4433 -> [_ _]
                          tunnel: w4432 -> [_ _]
                          tunnel: w4431 -> [_ w4473]
                          tunnel: w4430 -> [_ w4472]
                          tunnel: w4429 -> [_ w4437]
                          tunnel: w4426 -> [_ w4469]
                          tunnel: w4425 -> [_ w4468]
                          tunnel: w4424 -> [_ w4466]
                          tunnel: w4423 -> [_ w4458]
                          frame False {
                          }
                          frame True {
                            n2455 = local read "TDMS LAB03-2"() -> (w4471:refnum<k34>)
                            n2456 = Build Array(w4468) -> (w4463:dbl[])
                            n2457 = Build Array(w4466) -> (w4462:dbl[])
                            n2458 = Build Array(w4473) -> (w4461:dbl[])
                            n2459 = Build Array(w4474) -> (w4460:dbl[])
                            n2460 = Build Array(w4469) -> (w4465:dbl[])
                            n2461 = Build Array(w4467) -> (w4464:dbl[])
                            n2462 = Build Array(w4472) -> (w4459:dbl[])
                            n2463 = Build Array("AMPS ON", "AMPS OFF", "VOLTS", "PF", "TEMP Live", "TEMP Neut", "CYCLE") -> (w4442:string[])
                            n2464 = Bundle By Name("Y"=w4465, "t0"=w4458) -> (w4457:waveform(dbl))  [unwired: 1 in]
                            n2465 = Bundle By Name("Y"=w4464, "t0"=w4458) -> (w4456:waveform(dbl))  [unwired: 1 in]
                            n2466 = Bundle By Name("Y"=w4463, "t0"=w4458) -> (w4455:waveform(dbl))  [unwired: 1 in]
                            n2467 = Bundle By Name("Y"=w4462, "t0"=w4458) -> (w4454:waveform(dbl))  [unwired: 1 in]
                            n2468 = Bundle By Name("Y"=w4461, "t0"=w4458) -> (w4453:waveform(dbl))  [unwired: 1 in]
                            n2469 = Bundle By Name("Y"=w4460, "t0"=w4458) -> (w4452:waveform(dbl))  [unwired: 1 in]
                            n2470 = Bundle By Name("Y"=w4459, "t0"=w4458) -> (w4451:waveform(dbl))  [unwired: 1 in]
                            n2471 = Build Array(w4457, w4456, w4455, w4454, w4453, w4452, w4451) -> (w4450:waveform(dbl)[])
                            n2472 = TDMS Write(0:w4471, 5:"TEST VALUES", 7:w4442, 9:w4450) -> (4:w4441:refnum<k34>, 6:w4440:string, 15:w4439:errorcluster)  [unwired: 2 in, 1 out]
                            n2473 = TDMS Write(0:w4441, 5:w4440, 7:"TIME", 9:w4437, 11:w4439) -> (15:w4436:errorcluster)  [unwired: 1 in, 3 out]
                            n2474 = local write "data file error"(w4436) -> ()
                          }
                        }
                      }
                    }
                  }
                }
              }
              frame #6 {
                n2475 = case shown="True" w4475 {
                  tunnel: w4479 -> [_ w4484]
                  tunnel: w4478 -> [_ w4483]
                  tunnel: w4477 -> [_ w4481]
                  tunnel: w4476 -> [_ w4480]
                  frame False {
                  }
                  frame True {
                    n2476 = local read "DISP LAB04-1"() -> (w4485:T4)
                    n2477 = local read "SIG LAB04-1"() -> (w4486:T2)
                    n2478 = local read "ON L04-1"() -> (w4482:cluster{"amps":dbl, "volts":dbl, "pf":dbl})
                    n2479 = Unbundle(w4486) -> ("AMPS"=w4492:dbl, "VOLTS"=w4490:dbl, "PF"=w4489:dbl, "Tmp Live"=w4488:dbl, "Tmp Neut"=w4491:dbl)
                    n2480 = Unbundle(w4485) -> ("CYCLE"=w4487:dbl)  [unwired: 2 out]
                    n2481 = stacked-sequence {
                      tunnel: w4492 -> [w4496 w4515]
                      tunnel: w4491 -> [_ w4514]
                      tunnel: w4490 -> [w4495 w4513]
                      tunnel: w4489 -> [w4494 w4512]
                      tunnel: w4488 -> [_ w4511]
                      tunnel: w4487 -> [_ w4510]
                      tunnel: w4484 -> [_ w4509]
                      tunnel: w4483 -> [w4497 _]
                      tunnel: w4482 -> [w4493 w4507]
                      tunnel: w4481 -> [_ w4508]
                      tunnel: w4480 -> [_ w4503]
                      frame #0 {
                        n2482 = case shown="True" w4497 {
                          tunnel: w4496 -> [_ w4502]
                          tunnel: w4495 -> [_ w4501]
                          tunnel: w4494 -> [_ w4500]
                          tunnel: w4493 -> [_ w4498]
                          frame False {
                          }
                          frame True {
                            n2483 = Bundle(cluster=w4498, "amps"=w4502, "volts"=w4501, "pf"=w4500) -> (w4499:cluster{"amps":dbl, "volts":dbl, "pf":dbl})
                            n2484 = local write "ON L04-1"(w4499) -> ()
                          }
                        }
                      }
                      frame #1 {
                        n2485 = Unbundle(w4507) -> ("amps"=w4506:dbl, "volts"=w4505:dbl, "pf"=w4504:dbl)
                        n2486 = case shown="True" w4508 {
                          tunnel: w4515 -> [_ w4547]
                          tunnel: w4514 -> [_ w4554]
                          tunnel: w4513 -> [_ _]
                          tunnel: w4512 -> [_ _]
                          tunnel: w4511 -> [_ w4553]
                          tunnel: w4510 -> [_ w4552]
                          tunnel: w4509 -> [_ w4517]
                          tunnel: w4506 -> [_ w4549]
                          tunnel: w4505 -> [_ w4548]
                          tunnel: w4504 -> [_ w4546]
                          tunnel: w4503 -> [_ w4538]
                          frame False {
                          }
                          frame True {
                            n2487 = local read "TDMS LAB04-1"() -> (w4551:refnum<k34>)
                            n2488 = Build Array(w4548) -> (w4543:dbl[])
                            n2489 = Build Array(w4546) -> (w4542:dbl[])
                            n2490 = Build Array(w4553) -> (w4541:dbl[])
                            n2491 = Build Array(w4554) -> (w4540:dbl[])
                            n2492 = Build Array(w4549) -> (w4545:dbl[])
                            n2493 = Build Array(w4547) -> (w4544:dbl[])
                            n2494 = Build Array(w4552) -> (w4539:dbl[])
                            n2495 = Build Array("AMPS ON", "AMPS OFF", "VOLTS", "PF", "TEMP Live", "TEMP Neut", "CYCLE") -> (w4522:string[])
                            n2496 = Bundle By Name("Y"=w4545, "t0"=w4538) -> (w4537:waveform(dbl))  [unwired: 1 in]
                            n2497 = Bundle By Name("Y"=w4544, "t0"=w4538) -> (w4536:waveform(dbl))  [unwired: 1 in]
                            n2498 = Bundle By Name("Y"=w4543, "t0"=w4538) -> (w4535:waveform(dbl))  [unwired: 1 in]
                            n2499 = Bundle By Name("Y"=w4542, "t0"=w4538) -> (w4534:waveform(dbl))  [unwired: 1 in]
                            n2500 = Bundle By Name("Y"=w4541, "t0"=w4538) -> (w4533:waveform(dbl))  [unwired: 1 in]
                            n2501 = Bundle By Name("Y"=w4540, "t0"=w4538) -> (w4532:waveform(dbl))  [unwired: 1 in]
                            n2502 = Bundle By Name("Y"=w4539, "t0"=w4538) -> (w4531:waveform(dbl))  [unwired: 1 in]
                            n2503 = Build Array(w4537, w4536, w4535, w4534, w4533, w4532, w4531) -> (w4530:waveform(dbl)[])
                            n2504 = TDMS Write(0:w4551, 5:"TEST VALUES", 7:w4522, 9:w4530) -> (4:w4521:refnum<k34>, 6:w4520:string, 15:w4519:errorcluster)  [unwired: 2 in, 1 out]
                            n2505 = TDMS Write(0:w4521, 5:w4520, 7:"TIME", 9:w4517, 11:w4519) -> (15:w4516:errorcluster)  [unwired: 1 in, 3 out]
                            n2506 = local write "data file error"(w4516) -> ()
                          }
                        }
                      }
                    }
                  }
                }
              }
              frame #7 {
                n2507 = case shown="True" w4555 {
                  tunnel: w4559 -> [_ w4564]
                  tunnel: w4558 -> [_ w4563]
                  tunnel: w4557 -> [_ w4561]
                  tunnel: w4556 -> [_ w4560]
                  frame False {
                  }
                  frame True {
                    n2508 = local read "DISP LAB04-2"() -> (w4565:T4)
                    n2509 = local read "SIG LAB04-2"() -> (w4566:T2)
                    n2510 = local read "ON L04-2"() -> (w4562:cluster{"amps":dbl, "volts":dbl, "pf":dbl})
                    n2511 = Unbundle(w4566) -> ("AMPS"=w4572:dbl, "VOLTS"=w4570:dbl, "PF"=w4569:dbl, "Tmp Live"=w4568:dbl, "Tmp Neut"=w4571:dbl)
                    n2512 = Unbundle(w4565) -> ("CYCLE"=w4567:dbl)  [unwired: 2 out]
                    n2513 = stacked-sequence {
                      tunnel: w4572 -> [w4576 w4595]
                      tunnel: w4571 -> [_ w4594]
                      tunnel: w4570 -> [w4575 w4593]
                      tunnel: w4569 -> [w4574 w4592]
                      tunnel: w4568 -> [_ w4591]
                      tunnel: w4567 -> [_ w4590]
                      tunnel: w4564 -> [_ w4589]
                      tunnel: w4563 -> [w4577 _]
                      tunnel: w4562 -> [w4573 w4587]
                      tunnel: w4561 -> [_ w4588]
                      tunnel: w4560 -> [_ w4583]
                      frame #0 {
                        n2514 = case shown="True" w4577 {
                          tunnel: w4576 -> [_ w4582]
                          tunnel: w4575 -> [_ w4581]
                          tunnel: w4574 -> [_ w4580]
                          tunnel: w4573 -> [_ w4578]
                          frame False {
                          }
                          frame True {
                            n2515 = Bundle(cluster=w4578, "amps"=w4582, "volts"=w4581, "pf"=w4580) -> (w4579:cluster{"amps":dbl, "volts":dbl, "pf":dbl})
                            n2516 = local write "ON L04-2"(w4579) -> ()
                          }
                        }
                      }
                      frame #1 {
                        n2517 = Unbundle(w4587) -> ("amps"=w4586:dbl, "volts"=w4585:dbl, "pf"=w4584:dbl)
                        n2518 = case shown="True" w4588 {
                          tunnel: w4595 -> [_ w4627]
                          tunnel: w4594 -> [_ w4634]
                          tunnel: w4593 -> [_ _]
                          tunnel: w4592 -> [_ _]
                          tunnel: w4591 -> [_ w4633]
                          tunnel: w4590 -> [_ w4632]
                          tunnel: w4589 -> [_ w4597]
                          tunnel: w4586 -> [_ w4629]
                          tunnel: w4585 -> [_ w4628]
                          tunnel: w4584 -> [_ w4626]
                          tunnel: w4583 -> [_ w4618]
                          frame False {
                          }
                          frame True {
                            n2519 = local read "TDMS LAB04-2"() -> (w4631:refnum<k34>)
                            n2520 = Build Array(w4628) -> (w4623:dbl[])
                            n2521 = Build Array(w4626) -> (w4622:dbl[])
                            n2522 = Build Array(w4633) -> (w4621:dbl[])
                            n2523 = Build Array(w4634) -> (w4620:dbl[])
                            n2524 = Build Array(w4629) -> (w4625:dbl[])
                            n2525 = Build Array(w4627) -> (w4624:dbl[])
                            n2526 = Build Array(w4632) -> (w4619:dbl[])
                            n2527 = Build Array("AMPS ON", "AMPS OFF", "VOLTS", "PF", "TEMP Live", "TEMP Neut", "CYCLE") -> (w4602:string[])
                            n2528 = Bundle By Name("Y"=w4625, "t0"=w4618) -> (w4617:waveform(dbl))  [unwired: 1 in]
                            n2529 = Bundle By Name("Y"=w4624, "t0"=w4618) -> (w4616:waveform(dbl))  [unwired: 1 in]
                            n2530 = Bundle By Name("Y"=w4623, "t0"=w4618) -> (w4615:waveform(dbl))  [unwired: 1 in]
                            n2531 = Bundle By Name("Y"=w4622, "t0"=w4618) -> (w4614:waveform(dbl))  [unwired: 1 in]
                            n2532 = Bundle By Name("Y"=w4621, "t0"=w4618) -> (w4613:waveform(dbl))  [unwired: 1 in]
                            n2533 = Bundle By Name("Y"=w4620, "t0"=w4618) -> (w4612:waveform(dbl))  [unwired: 1 in]
                            n2534 = Bundle By Name("Y"=w4619, "t0"=w4618) -> (w4611:waveform(dbl))  [unwired: 1 in]
                            n2535 = Build Array(w4617, w4616, w4615, w4614, w4613, w4612, w4611) -> (w4610:waveform(dbl)[])
                            n2536 = TDMS Write(0:w4631, 5:"TEST VALUES", 7:w4602, 9:w4610) -> (4:w4601:refnum<k34>, 6:w4600:string, 15:w4599:errorcluster)  [unwired: 2 in, 1 out]
                            n2537 = TDMS Write(0:w4601, 5:w4600, 7:"TIME", 9:w4597, 11:w4599) -> (15:w4596:errorcluster)  [unwired: 1 in, 3 out]
